vi "FPGA.vi"() -> ()   [LabVIEW 2015]
uses:
  <vilib>/Platform/TimedLoop/XDataNode/timing_clust.ctl
  <vilib>/Platform/TimedLoop/XDataNode/nitl_modes.ctl
  <vilib>/Platform/TimedLoop/XDataNode/wakeup.ctl
  <vilib>/rvi/Emulation/niFpgaGetClockAttributes.vi
  <vilib>/rvi/Emulation/niFpgaSctlEmulationGetInTimedLoop.vi
  <vilib>/rvi/Emulation/niFpgaEmulationReportErrorSimple.vi
  <vilib>/rvi/eio/common/nirviEmuTemplateMethod_errors.vi
  <vilib>/rvi/Emulation/niFpgaCriticalErrorInLSC.vi
  <vilib>/rvi/Emulation/niFpgaEmulationIsFPGAContextNoSignature.vi
  <vilib>/rvi/DataTransferAndStorage/Container/Common/niFpgaContainerGetUniqueNameForEmu.vi
  <vilib>/rvi/Memory/Memory_Emulation/niFpgaMemoryEmulationCacheClearOnFirstRun.vi
  <vilib>/rvi/Memory/Memory_Emulation/nirvimemoryEmulationManagerCache_MakeExclusive.vi
  <vilib>/rvi/Memory/Memory_Emulation/niFpgaMemoryEmulationValidateCache.vi
  <vilib>/rvi/Memory/Memory_Emulation/nirvimemoryEmulationManagerCache_InsertValue.vi
  <vilib>/Utility/error.llb/Clear Errors.vi
  <vilib>/rvi/Memory/Memory_Emulation/nirvimemoryEmulationManagerCache_ReleaseExclusive.vi
  <vilib>/rvi/Memory/Memory_Emulation/nirvimemoryEmulationManagerCache_GetValue.vi
  <vilib>/rvi/Memory/Memory_Emulation/nirvimemoryEmulationManagerCache_SetValue.vi
  <vilib>/rvi/Emulation/niFpgaProcessEmulError.vi
  <vilib>/rvi/Memory/Memory_Emulation/nirvimemoryFastEmulation.vi
  <vilib>/rvi/Memory/Memory_Emulation/nirvimemoryEmulation.vi
  <vilib>/rvi/errors/nirviReportUnexpectedCaseInternalError (U32).vi
  <vilib>/eio/EIONode/EIONode.xnode
  <vilib>/Platform/TimedLoop/XDataNode/XDataNode.xnode
  <vilib>/rvi/DataTransferAndStorage/Container/XNode/niFpgaContainer.xnode
  <vilib>/rvi/DataTransferAndStorage/Register/Emulation/niFpgaRegisterEmulation.vi
  <vilib>/Platform/TimedLoop/XDataNode/XDNodeRunTimeDep.lvlib
panel:
  in  "Амплитуда (0-4096)":u16=4096
  out "Принимаемые\nданные":u16[](array[numeric]) format="%04x"
  out "Ошибка \nпередачи на ОУ":bool
  out "Ошибка \nчтения из ОУ":bool
  in  "RX":bool
  out "TX":bool
  in  "Передаваемые данные":u16[](array[numeric])=[4, 821, 65535, 13380, 0, 0, 0, 0, 0, 0, 0, 0, 0, 0, 0, 0, 0, 0, 0, 0, 0, 0, 0, 0, 0, 0, 0, 0, 0, 0, 0, 0, 0, 0] format="%04x"
  in  "Кол-во слов \nдля приема":u8=4
  in  "Кол-во слов \nдля передачи":u8=1
  in  "адрес ОУ (0-30)":u8=8
  in  "Подадрес (1-30)":u8=4
  in  "Команда управления":T1(ring)=enum."Блокировать передатчик"
  in  "Отправить\nRx CMD":bool
  in  "Отправить\nTx CMD":bool
  in  "Отправить команду ОУ":bool
  out "Машина состояний КШ":T2
  # "Тестовая панель контроллера шины  MIL STD 1553"
  # "Настройки"
  # "Команда передачи:"
  # "Управление ОУ:"
  # "Команда чтения:"
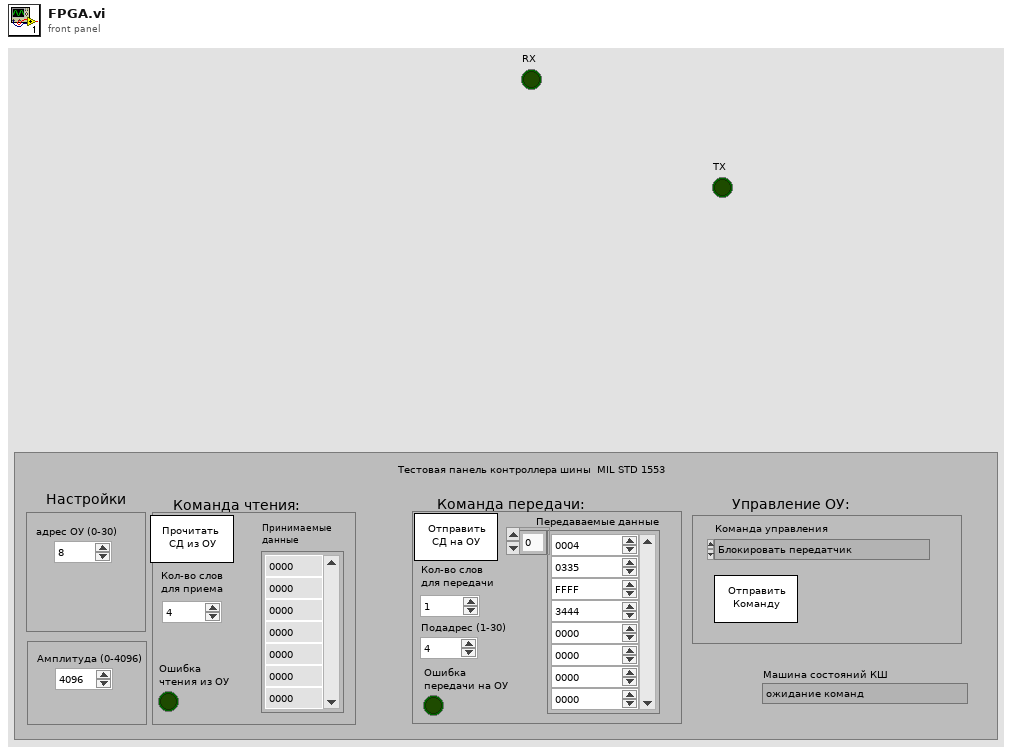
[diagram p1: front panel]
types:
  T1 = enum16{"Принять управление интерфейсом", "Синхронизация", "Передать ОС", "Начать самоконтроль ОУ", "Блокировать передатчик", "Разблокировать передатчик", "Блокировать признак неисправности ОУ", "Разблокировать признак неисправнотси ОУ", "Установить ОУ в исходное состояние", "Резерв", "Передать векорное слово", "Синхронизвция с СД", "Передать последнюю команду", "Передать слово ВСК ОУ", "Блокировать i-й передатчик", "Разблокировать i-й передатчик", "Резерв 2"}
  T2 = typedef "машина состояний КШ.ctl" = enum16{"ожидание команд", "Подготовка команды RX", "Подготовка команды TX", "кодер манчестер КС", "таймаут t2 между словами", "Передача", "ожидание rising СД", "замер длительности true СД", "чтение бит СД", "манчестер декодер СД", "чтение СД", "ожидание rising ОС", "замер длительности false ОС", "замер длительности true OC", "чтение бит ОС", "манчестер декодер ОС", "чтение ОС", "подготовка СД", "кодирование СД", "отправка СД"}
  T3 = typedef "XDNodeRunTimeDep.lvlib/timing_clust.ctl" = cluster{"Expected End [f-1]":u64, "Actual End [f-1]":u64, "Finished Late? [f-1]":bool, "Expected End [i-1]":u64, "Actual End [i-1]":u64, "Finished Late? [i-1]":bool, "Expected Start [i]":u64, "Actual Start [i]":u64, "Expected Start [f]":u64, "Actual Start [f]":u64, "Source Name":string, "Structure Name":string, "Period":i64, "Deadline":i64, "Offset":i64, "Start":i64, "Priority":i32, "Timeout":i32, "Mode":T4, "Wakeup Reason":T5, "Error":errorcluster, "Source Type":string, "Secondary Source Type":string, "Global End Time":u64, "Global Start Time":u64, "Frame Duration":u64, "Iteration Duration":u64, "Assigned CPU":i32, "I/O Scan Engine Mode":u32}
  T4 = typedef "XDNodeRunTimeDep.lvlib/nitl_modes.ctl" = enum32{"No Change", "Process missed periods, maintain original phase", "Discard missed periods, maintain original phase", "Process missed periods, ignore original phase", "Discard missed periods, ignore original phase"}
  T5 = typedef "XDNodeRunTimeDep.lvlib/wakeup.ctl" = enum32{"Normal", "Aborted", "Asynchronous wakeup", "Timing source error", "Timed loop error", "Timeout"}
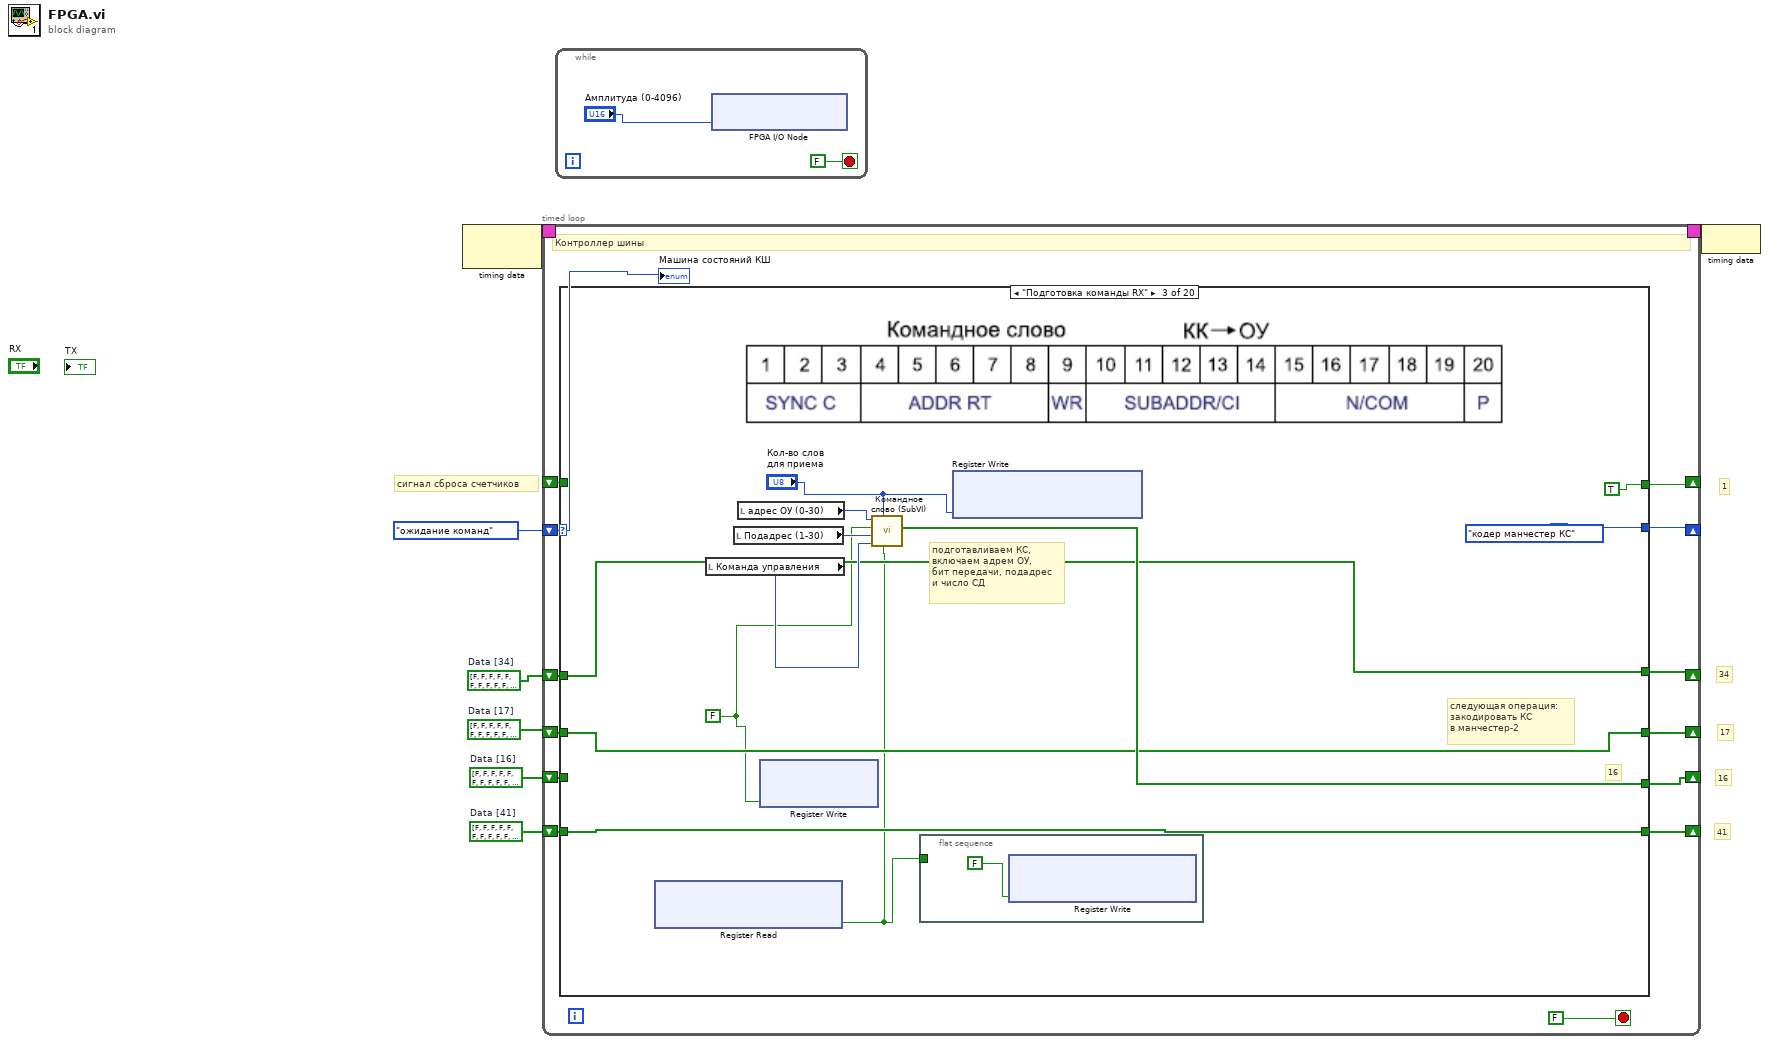
[diagram p0: block diagram]
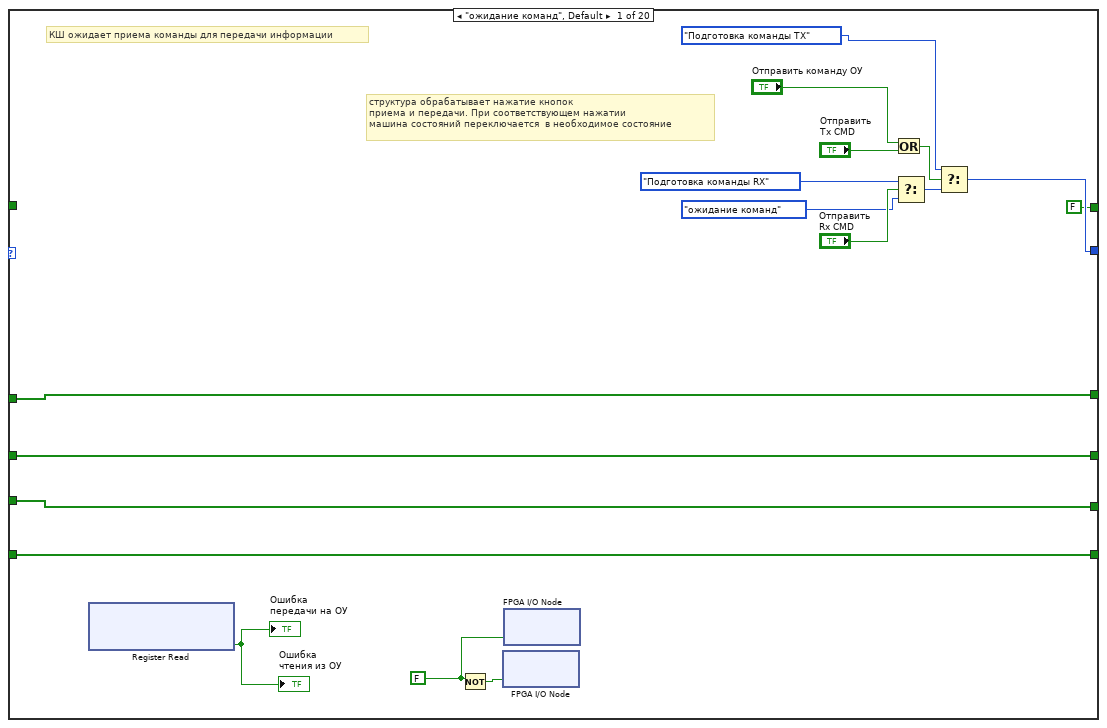
[diagram p2: hidden frame]
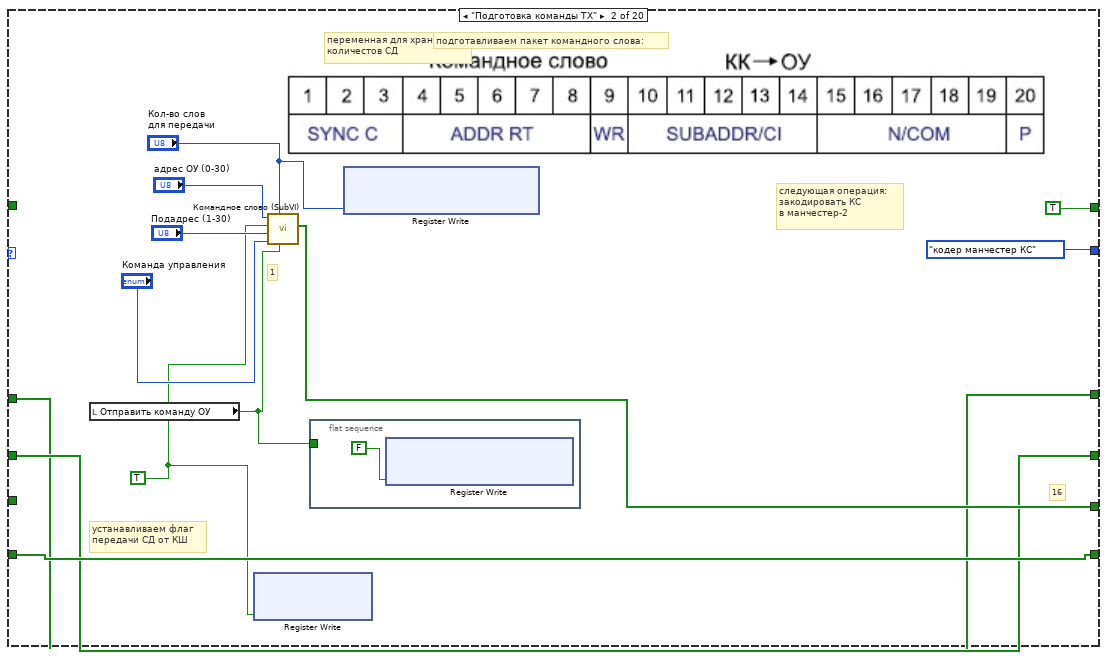
[diagram p3: hidden frame]
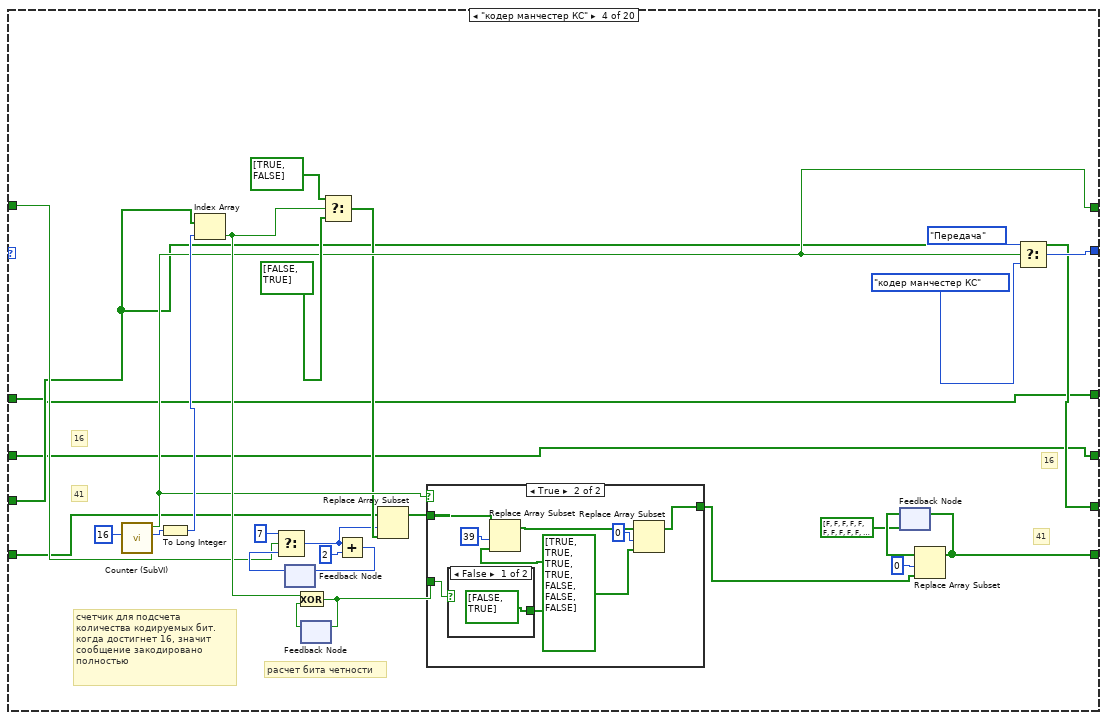
[diagram p4: hidden frame]
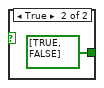
[diagram p6: hidden frame]
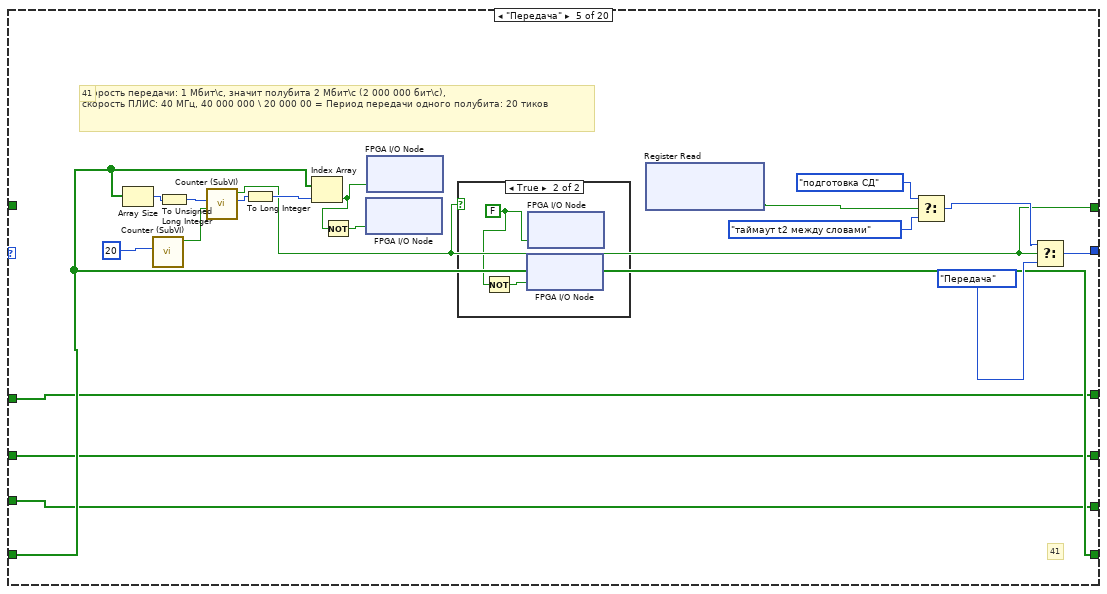
[diagram p7: hidden frame]
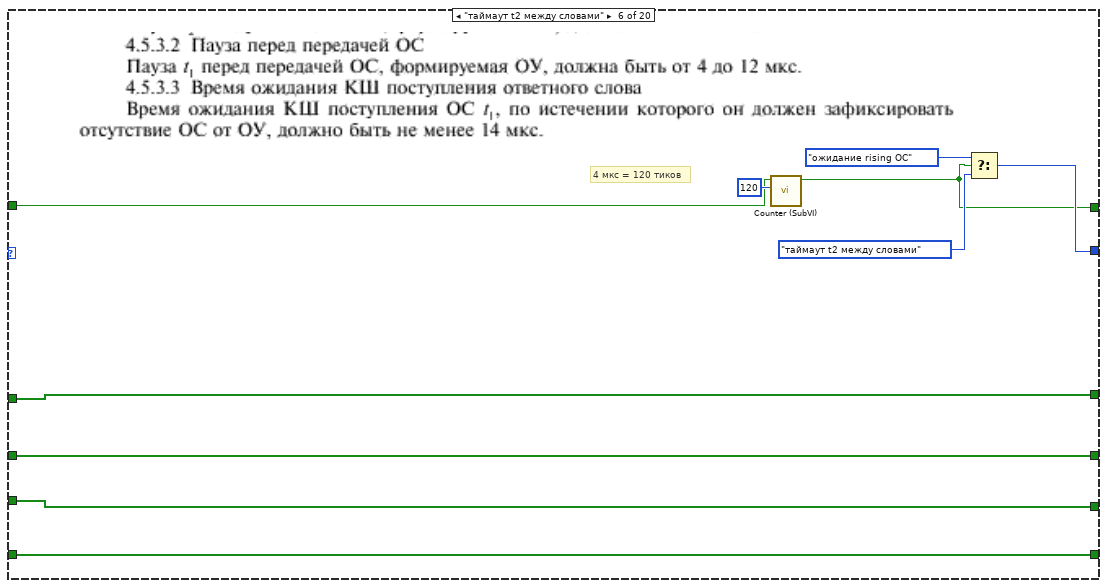
[diagram p9: hidden frame]
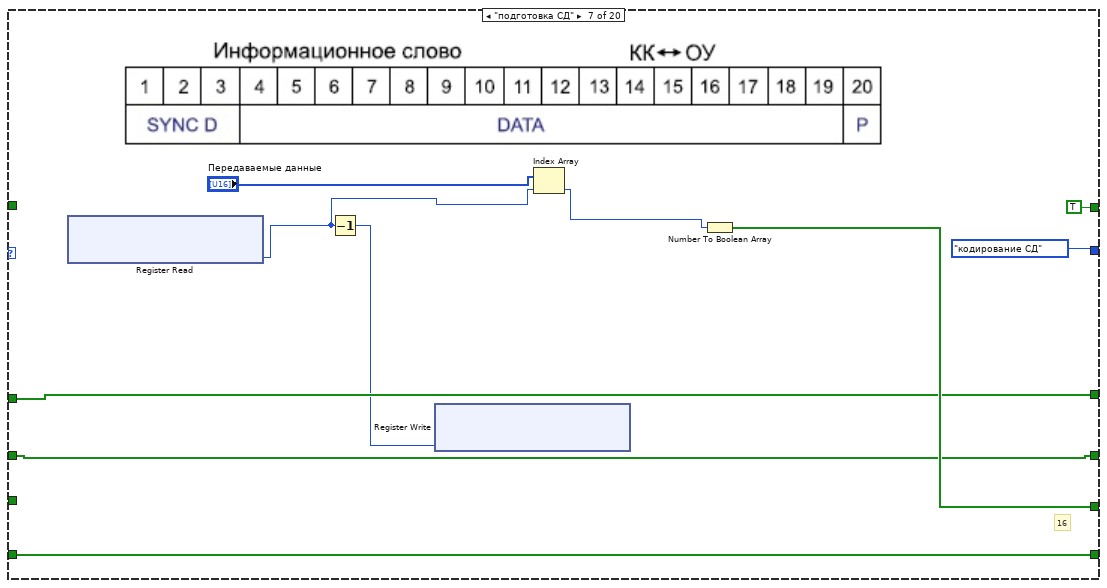
[diagram p10: hidden frame]
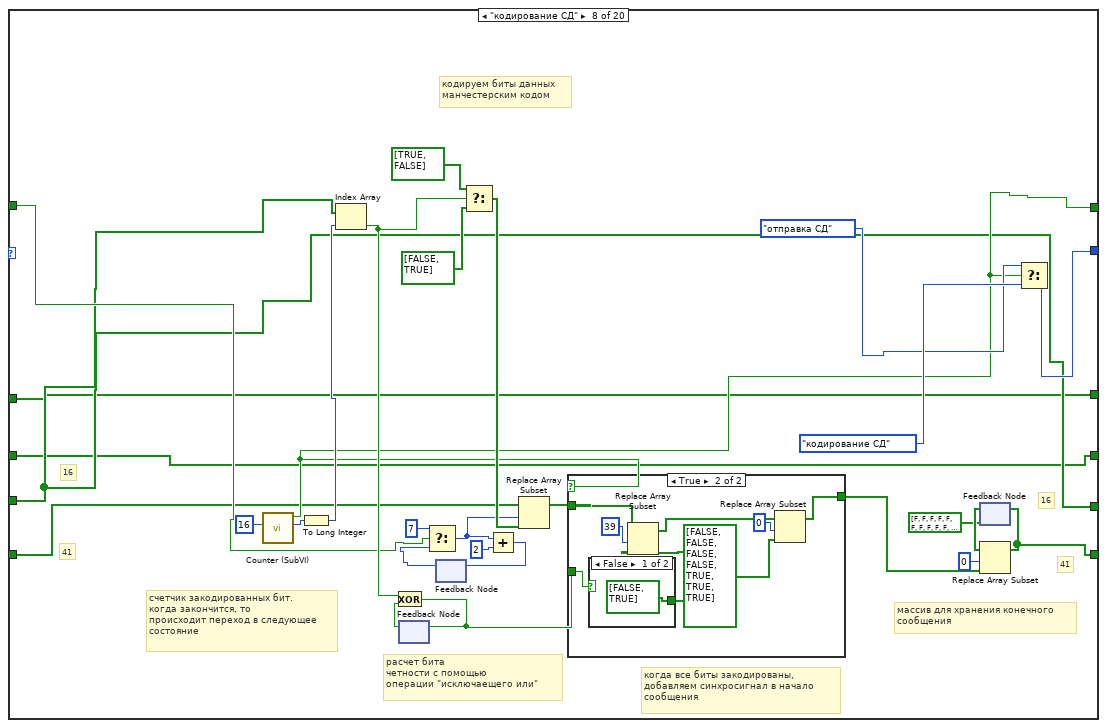
[diagram p11: hidden frame]
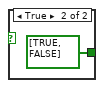
[diagram p13: hidden frame]
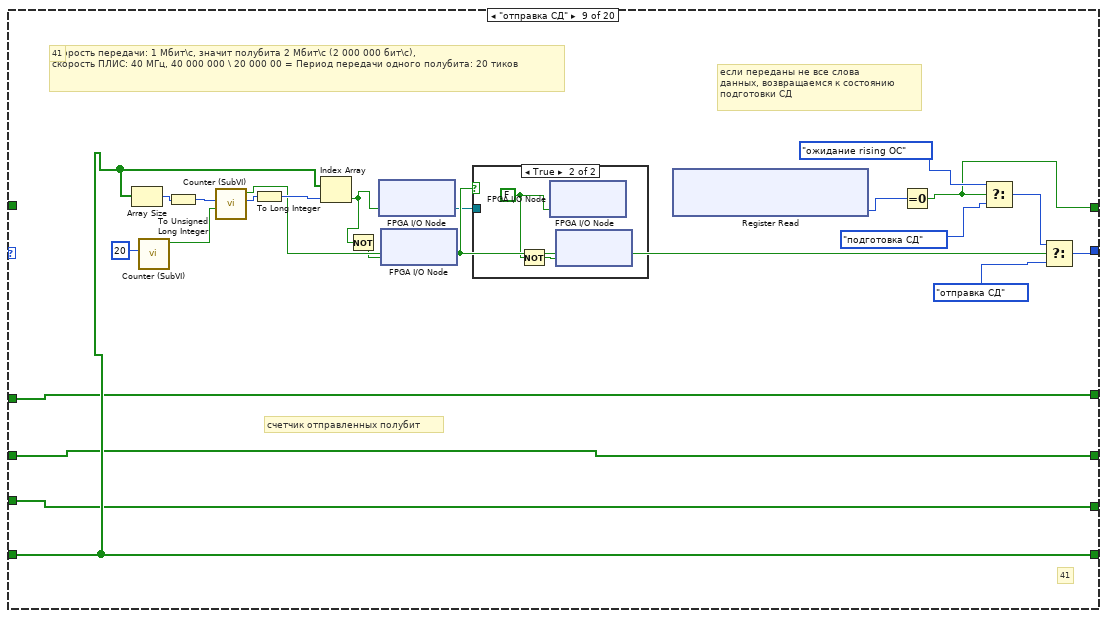
[diagram p14: hidden frame]
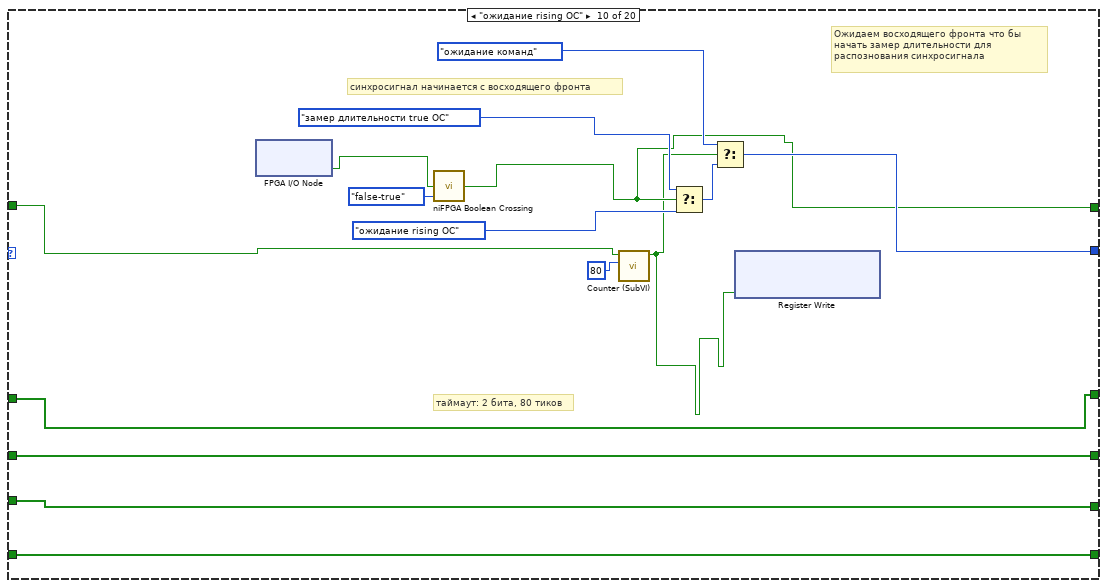
[diagram p16: hidden frame]
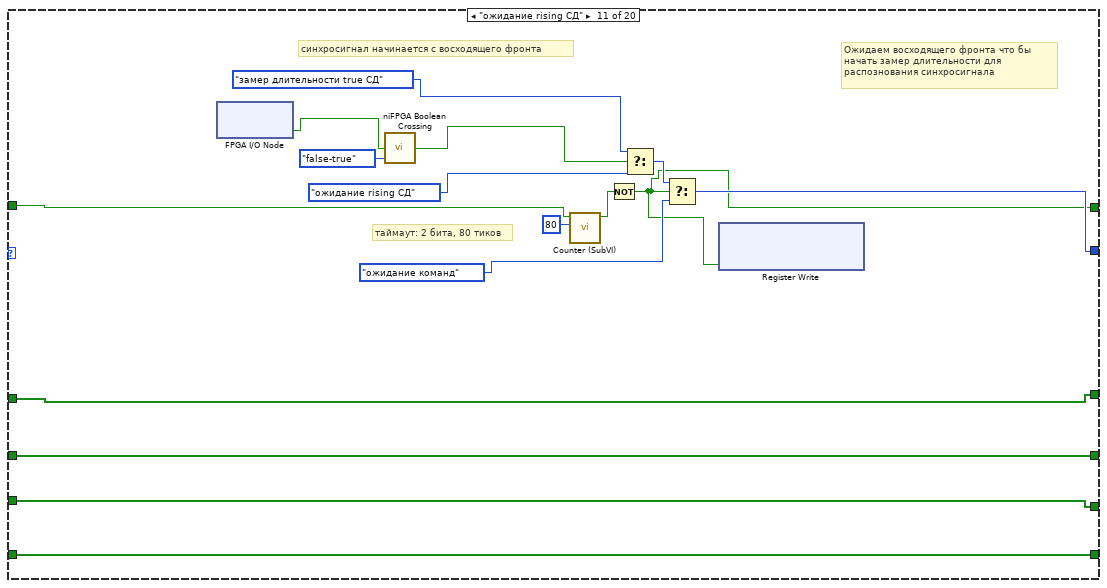
[diagram p17: hidden frame]
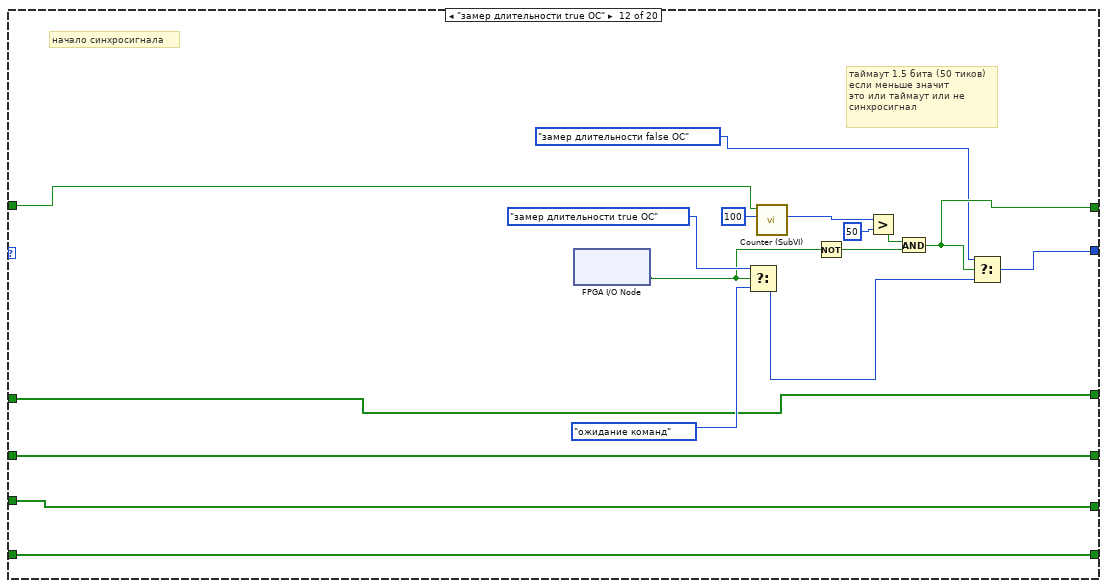
[diagram p18: hidden frame]
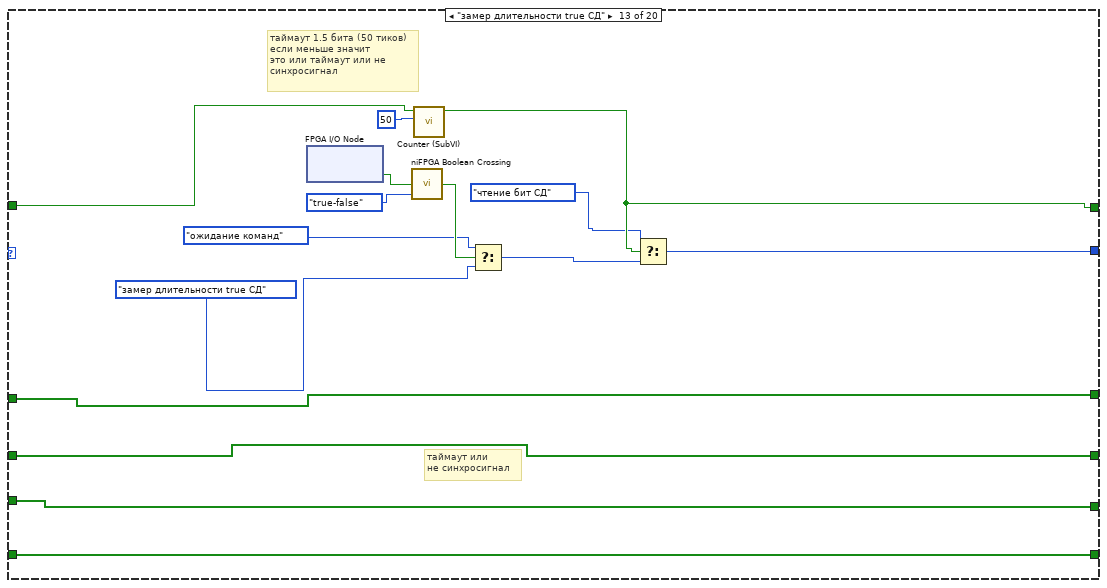
[diagram p19: hidden frame]
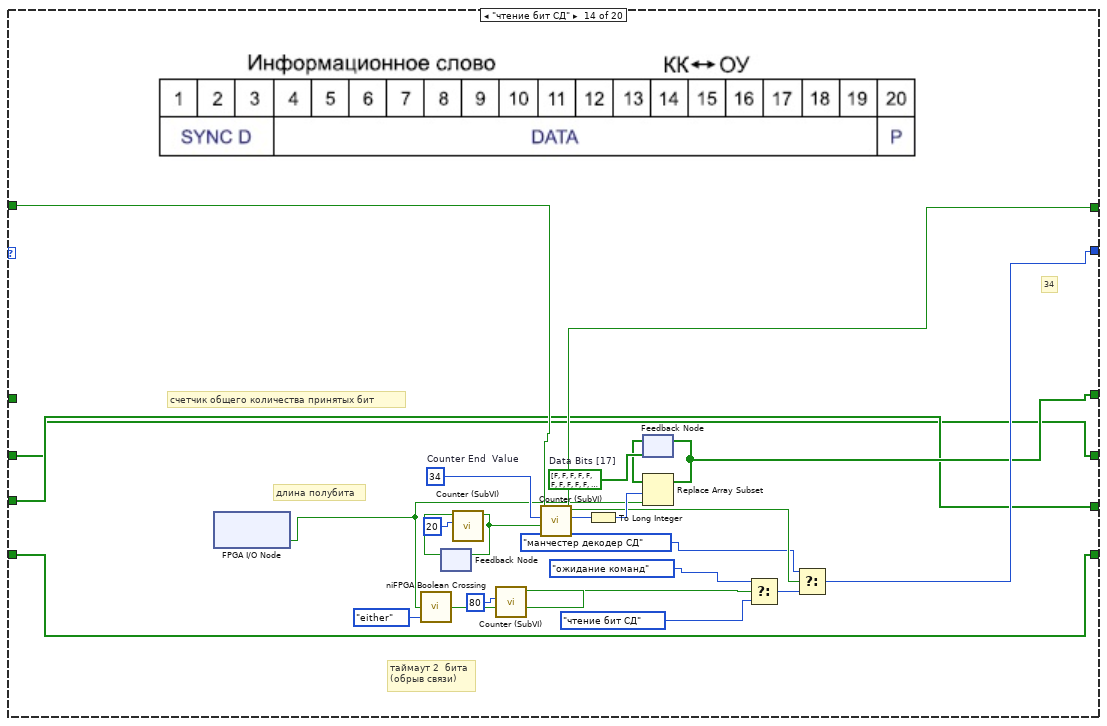
[diagram p20: hidden frame]
diagram:
  w3 = bool[] [FALSE, FALSE, FALSE, FALSE, FALSE, FALSE, FALSE, FALSE, FALSE, FALSE, FALSE, FALSE, FALSE, FALSE, FALSE, FALSE, FALSE, FALSE, FALSE, FALSE, FALSE, FALSE, FALSE, FALSE, FALSE, FALSE, FALSE, FALSE, FALSE, FALSE, FALSE, FALSE, FALSE, FALSE, FALSE, FALSE, FALSE, FALSE, FALSE, FALSE, FALSE]  # Data [41]
  w4 = bool[] [FALSE, FALSE, FALSE, FALSE, FALSE, FALSE, FALSE, FALSE, FALSE, FALSE, FALSE, FALSE, FALSE, FALSE, FALSE, FALSE]  # Data [16]
  w5 = bool[] [FALSE, FALSE, FALSE, FALSE, FALSE, FALSE, FALSE, FALSE, FALSE, FALSE, FALSE, FALSE, FALSE, FALSE, FALSE, FALSE, FALSE]  # Data [17]
  w6 = bool[] [FALSE, FALSE, FALSE, FALSE, FALSE, FALSE, FALSE, FALSE, FALSE, FALSE, FALSE, FALSE, FALSE, FALSE, FALSE, FALSE, FALSE, FALSE, FALSE, FALSE, FALSE, FALSE, FALSE, FALSE, FALSE, FALSE, FALSE, FALSE, FALSE, FALSE, FALSE, FALSE, FALSE, FALSE]  # Data [34]
  # "1"
  # "34"
  # "41"
  # "17"
  # "16"
  # "сигнал сброса счетчиков"
  n1 = node-c288() -> (w2:T3)  [unwired: 1 in]
  n2 = timed-loop {
    shift-right: [w19] -> _
    shift-left: машина_состояний_КШ."ожидание команд" ("Машина состояний КШ") -> [w12]
    shift-right: [w18] -> _
    shift-left: _ -> [w17]
    shift-right: [w16] -> _
    shift-left: w6 -> [w15]
    shift-right: [w14] -> _
    shift-left: w5 -> [w13]
    shift-right: [w8] -> _
    shift-left: w4 -> [w10]
    shift-right: [w9] -> _
    shift-left: w3 -> [w11]
    timing: w2 -> [_]
    timing-out: [_] -> w1
    stop <- FALSE stop-if-true
    # "Контроллер шины"
    n3 = case shown="\"Подготовка команды RX\"" w12 {
      tunnel: [w36 машина_состояний_КШ."кодер манчестер КС" ("Машина состояний КШ") машина_состояний_КШ."кодер манчестер КС" ("Машина состояний КШ") w83 w118 w133 машина_состояний_КШ."кодирование СД" ("Машина состояний КШ") w162 w194 w221 w235 w249 w264 w280 w316 w338 w349 w362 w400 w416] -> w19
      tunnel: [FALSE ("End Reached") TRUE ("End Reached") TRUE ("End Reached") w80 w111 w129 TRUE ("End Reached") w150 w193 w215 w223 w248 w265 w281 FALSE ("End Reached") FALSE ("End Reached") w348 w364 FALSE ("End Reached") FALSE ("End Reached")] -> w18
      tunnel: w17 -> [_ _ _ w70 _ w130 _ w152 _ w214 w233 w250 w266 w279 w307 _ w350 w365 w392 _]
      tunnel: [w25 w40 w54 w65 w107 w128 w139 w145 w189 w210 w226 w240 w257 w278 w312 w329 w341 w363 w387 w410] -> w16
      tunnel: w15 -> [w25 w40 w54 w65 w107 w128 w139 w145 w189 w210 w226 w240 w257 _ w312 w329 w341 _ w387 w410]
      tunnel: [w26 w41 w55 w64 w108 w127 w140 w146 w190 w211 w227 w241 w258 w272 w315 w330 w342 w356 w399 w411] -> w14
      tunnel: w13 -> [w26 w41 w55 w64 w108 w127 w140 w146 w190 w211 w227 w241 w258 w272 _ w330 w342 w356 _ w411]
      tunnel: w11 -> [w28 w42 w56 w67 w110 w125 w141 w149 w192 w213 w229 w243 w260 w274 w306 w332 w344 w358 w391 w413]
      tunnel: w10 -> [w27 _ _ w66 w109 w126 _ w147 w191 w212 w228 w242 w259 w273 w305 w331 w343 w357 w390 w412]
      tunnel: [w28 w42 w56 w68 w110 w125 w141 w148 w192 w213 w229 w243 w260 w274 w306 w332 w344 w358 w391 w413] -> w9
      tunnel: [w27 w43 w57 w66 w109 w126 w142 w147 w191 w212 w228 w242 w259 w273 w305 w331 w343 w357 w390 w412] -> w8
      frame "ожидание команд", Default {
        w21 = FALSE ("TX")
        # "структура обрабатывает нажатие кнопок \nприема и передачи. При соответствующем нажатии\nмашина состояний переключается  в необходимое состояние"
        # "КШ ожидает приема команды для передачи информации"
        n4 = xnode ("Register Read")() -> ("Data"=→"Ошибка \nчтения из ОУ" →"Ошибка \nпередачи на ОУ":bool)  [unwired: 1 in, 1 out]
        n5 = Not(x=w21) -> (.not. x?=w22:bool)
        n6 = xnode "FPGA I/O Node"("TXinv"=w22) -> ()  [unwired: 1 in, 1 out]
        n7 = xnode "FPGA I/O Node"("TX"=w21) -> ()  [unwired: 1 in, 1 out]
        n8 = Or(x="Отправить команду ОУ", y="Отправить\nTx CMD") -> (x .or. y?=w32:bool)
        n9 = Select(t=машина_состояний_КШ."Подготовка команды RX" ("Машина состояний КШ"), s="Отправить\nRx CMD", f=машина_состояний_КШ."ожидание команд" ("Машина состояний КШ")) -> (s? t:f=w35:T2)
        n10 = Select(t=машина_состояний_КШ."Подготовка команды TX" ("Машина состояний КШ"), s=w32, f=w35) -> (s? t:f=w36:T2)
      }
      frame "Подготовка команды TX" {
        w39 = TRUE ("Разряд прием\\передача")
        # "16"
        # "устанавливаем флаг\nпередачи СД от КШ"
        # "следующая операция:\nзакодировать КС\nв манчестер-2"
        # "переменная для хранения\nколичестов СД"
        # "1"
        # "подготавливаем пакет командного слова:"
        n11 = local read "Отправить команду ОУ"() -> (w46:bool)
        n12 = xnode ("Register Write")("Data"=w39) -> ()  [unwired: 1 in, 1 out]
        n13 = call "Командное слово (SubVI).vi"("Признак команды"=w46, "Кол-во слов (1-32)"="Кол-во слов \nдля передачи", "Команда управления"="Команда управления", "Подадрес (1-30)"="Подадрес (1-30)", "Разряд прием\\передача"=w39, "адрес ОУ (0-30)"="адрес ОУ (0-30)") -> ("КС"=w43:bool[])  [unwired: 5 in]
        n14 = flat-sequence {
          tunnel: w46 -> [_]
          frame #0 {
            n15 = xnode ("Register Write")("Data"=FALSE ("Отправить команду ОУ")) -> ()  [unwired: 1 in, 1 out]
          }
        }
        n16 = xnode ("Register Write")("Data"="Кол-во слов \nдля передачи") -> ()  [unwired: 1 in, 1 out]
      }
      frame "Подготовка команды RX" {
        w53 = FALSE ("Разряд прием\\передача 2")
        # "16"
        # "следующая операция:\nзакодировать КС\nв манчестер-2"
        # "подготавливаем КС,\nвключаем адрем ОУ,\nбит передачи, подадрес\nи число СД"
        n17 = xnode ("Register Read")() -> ("Data"=w52:bool)  [unwired: 1 in, 1 out]
        n18 = local read "Команда управления"() -> (w60:T1)
        n19 = local read "Подадрес (1-30)"() -> (w61:u8)
        n20 = local read "адрес ОУ (0-30)"() -> (w62:u8)
        n21 = xnode ("Register Write")("Data"=w53) -> ()  [unwired: 1 in, 1 out]
        n22 = call "Командное слово (SubVI).vi"("Признак команды"=w52, "Кол-во слов (1-32)"="Кол-во слов \nдля приема", "Команда управления"=w60, "Подадрес (1-30)"=w61, "Разряд прием\\передача"=w53, "адрес ОУ (0-30)"=w62) -> ("КС"=w57:bool[])  [unwired: 5 in]
        n23 = flat-sequence {
          tunnel: w52 -> [_]
          frame #0 {
            n24 = xnode ("Register Write")("Data"=FALSE ("Отправить команду ОУ")) -> ()  [unwired: 1 in, 1 out]
          }
        }
        n25 = xnode ("Register Write")("Data"="Кол-во слов \nдля приема") -> ()  [unwired: 1 in, 1 out]
      }
      frame "кодер манчестер КС" {
        # "16"
        # "41"
        # "41"
        # "16"
        # "расчет бита четности"
        # "счетчик для подсчета\nколичества кодируемых бит.\nкогда достигнет 16, значит\nсообщение закодировано \nполностью"
        n26 = call "Counter (SubVI).vi"("Counter End  Value"=u32 16) -> ("Counter Value"=w86:u32, "End Reached"=w80:bool)  [unwired: 9 in]
        n27 = To Long Integer(number=w86) -> (32bit integer=w89:i32)
        n28 = Index Array(array=w66, index=w89) -> (element=w91:bool)
        n29 = feedback #1() -> (w72:i32)  [unwired: 1 in]
        n30 = Select(t=7 ("length"), s=w70, f=w72) -> (s? t:f=w69:i32)
        n31 = feedback #2() -> (w90:bool)  [unwired: 1 in]
        n32 = Exclusive Or(1:w90, 2:w91) -> (0:w92:bool)
        n33 = feedback-in #2(w92) -> ()
        n34 = Select(t=bool[] [TRUE, FALSE], s=w91, f=bool[] [FALSE, TRUE]) -> (s? t:f=w75:bool[])
        n35 = Add(x=w69, y=2 ("length")) -> (x+y=w73:i32)
        n36 = feedback-in #1(w73) -> ()
        n37 = Replace Array Subset(array=w67, new element=w75, index=w69) -> (w88:bool[])
        n38 = case shown="True" w80 {
          tunnel: w88 -> [w93 w99]
          tunnel: [w93 w100] -> w77
          tunnel: w92 -> [_ w96]
          frame False {
          }
          frame True {
            n39 = case shown="False" w96 {
              tunnel: [bool[] [FALSE, TRUE] bool[] [TRUE, FALSE]] -> w95
              frame False {
              }
              frame True {
              }
            }
            n40 = Replace Array Subset(array=w99, new element=w95, index=39) -> (w98:bool[])
            n41 = Replace Array Subset(array=w98, new element=bool[] [TRUE, TRUE, TRUE, TRUE, FALSE, FALSE, FALSE], index=0) -> (w100:bool[])
          }
        }
        n42 = feedback #3(bool[] [FALSE, FALSE, FALSE, FALSE, FALSE, FALSE, FALSE, FALSE, FALSE, FALSE, FALSE, FALSE, FALSE, FALSE, FALSE, FALSE, FALSE, FALSE, FALSE, FALSE, FALSE, FALSE, FALSE, FALSE, FALSE, FALSE, FALSE, FALSE, FALSE, FALSE, FALSE, FALSE, FALSE, FALSE, FALSE, FALSE, FALSE, FALSE, FALSE, FALSE, FALSE]) -> (w79:bool[])
        n43 = Replace Array Subset(array=w79, new element=w77, index=0) -> (w68:bool[])
        n44 = feedback-in #3(w68) -> ()
        n45 = Select(t=машина_состояний_КШ."Передача" ("Машина состояний КШ"), s=w80, f=машина_состояний_КШ."кодер манчестер КС" ("Машина состояний КШ")) -> (s? t:f=w83:T2)
      }
      frame "Передача" {
        # "скорость передачи: 1 Мбит\\с, значит полубита 2 Мбит\\с (2 000 000 бит\\с),\nскорость ПЛИС: 40 МГц, 40 000 000 \\ 20 000 00 = Период передачи одного полубита: 20 тиков"
        # "41"
        # "41"
        n46 = Array Size(array=w110) -> (size(s)=w116:i32)
        n47 = call "Counter (SubVI).vi"("Counter End  Value"=u32 20) -> ("End Reached"=w119:bool)  [unwired: 9 in, 1 out]
        n48 = To Unsigned Long Integer(number=w116) -> (unsigned 32bit integer=w115:u32)
        n49 = call "Counter (SubVI).vi"("Input Valid"=w119, "Counter End  Value"=w115) -> ("Counter Value"=w122:u32, "End Reached"=w111:bool)  [unwired: 8 in]
        n50 = To Long Integer(number=w122) -> (32bit integer=w121:i32)
        n51 = Index Array(array=w110, index=w121) -> (element=w104:bool)
        n52 = Not(x=w104) -> (.not. x?=w105:bool)
        n53 = xnode "FPGA I/O Node"("TXinv"=w105) -> ()  [unwired: 1 in, 1 out]
        n54 = xnode "FPGA I/O Node"("TX"=w104) -> ()  [unwired: 1 in, 1 out]
        n55 = case shown="True" w111 {
          frame False {
          }
          frame True {
            w123 = FALSE ("TX")
            n56 = Not(x=w123) -> (.not. x?=w124:bool)
            n57 = xnode "FPGA I/O Node"("TXinv"=w124) -> ()  [unwired: 1 in, 1 out]
            n58 = xnode "FPGA I/O Node"("TX"=w123) -> ()  [unwired: 1 in, 1 out]
          }
        }
        n59 = xnode ("Register Read")() -> ("Data"=w106:bool)  [unwired: 1 in, 1 out]
        n60 = Select(t=машина_состояний_КШ."подготовка СД" ("Машина состояний КШ"), s=w106, f=машина_состояний_КШ."таймаут t2 между словами" ("Машина состояний КШ")) -> (s? t:f=w113:T2)
        n61 = Select(t=w113, s=w111, f=машина_состояний_КШ."Передача" ("Машина состояний КШ")) -> (s? t:f=w118:T2)
      }
      frame "таймаут t2 между словами" {
        # "4 мкс = 120 тиков"
        n62 = call "Counter (SubVI).vi"("Counter End  Value"=u32 120, "Reset"=w130) -> ("End Reached"=w129:bool)  [unwired: 8 in, 1 out]
        n63 = Select(t=машина_состояний_КШ."ожидание rising ОС" ("Машина состояний КШ"), s=w129, f=машина_состояний_КШ."таймаут t2 между словами" ("Машина состояний КШ")) -> (s? t:f=w133:T2)
      }
      frame "подготовка СД" {
        # "16"
        n64 = xnode ("Register Read")() -> ("Data"=w136:u8)  [unwired: 1 in, 1 out]
        n65 = Decrement(x=w136) -> (x-1=w138:u8)
        n66 = xnode ("Register Write")("Data"=w138) -> ()  [unwired: 1 in, 1 out]
        n67 = Index Array(array="Передаваемые данные", index=w136) -> (element=w135:u16)
        n68 = Number To Boolean Array(number=w135) -> (Boolean array=w142:bool[])
      }
      frame "кодирование СД" {
        # "массив для хранения конечного\nсообщения"
        # "кодируем биты данных\nманчестерским кодом"
        # "когда все биты закодированы,\nдобавляем синхросигнал в начало \nсообщения"
        # "расчет бита\nчетности с помощью\nоперации \"исключаещего или\""
        # "счетчик закодированных бит.\nкогда закончится, то \nпроисходит переход в следующее\nсостояние"
        # "16"
        # "41"
        # "41"
        # "16"
        n69 = call "Counter (SubVI).vi"("Counter End  Value"=u32 16) -> ("Counter Value"=w167:u32, "End Reached"=w150:bool)  [unwired: 9 in]
        n70 = To Long Integer(number=w167) -> (32bit integer=w170:i32)
        n71 = Index Array(array=w147, index=w170) -> (element=w172:bool)
        n72 = feedback #4() -> (w171:bool)  [unwired: 1 in]
        n73 = Exclusive Or(1:w171, 2:w172) -> (0:w173:bool)
        n74 = feedback-in #4(w173) -> ()
        n75 = feedback #5() -> (w156:i32)  [unwired: 1 in]
        n76 = Select(t=7 ("length"), s=w152, f=w156) -> (s? t:f=w151:i32)
        n77 = Select(t=bool[] [TRUE, FALSE], s=w172, f=bool[] [FALSE, TRUE]) -> (s? t:f=w157:bool[])
        n78 = Add(x=w151, y=2 ("length")) -> (x+y=w154:i32)
        n79 = feedback-in #5(w154) -> ()
        n80 = Replace Array Subset(array=w149, new element=w157, index=w151) -> (w169:bool[])
        n81 = case shown="True" w150 {
          tunnel: w169 -> [w174 w180]
          tunnel: [w174 w181] -> w158
          tunnel: w173 -> [_ w177]
          frame False {
          }
          frame True {
            n82 = case shown="False" w177 {
              tunnel: [bool[] [FALSE, TRUE] bool[] [TRUE, FALSE]] -> w176
              frame False {
              }
              frame True {
              }
            }
            n83 = Replace Array Subset(array=w180, new element=w176, index=39) -> (w179:bool[])
            n84 = Replace Array Subset(array=w179, new element=bool[] [FALSE, FALSE, FALSE, FALSE, TRUE, TRUE, TRUE], index=0) -> (w181:bool[])
          }
        }
        n85 = feedback #6(bool[] [FALSE, FALSE, FALSE, FALSE, FALSE, FALSE, FALSE, FALSE, FALSE, FALSE, FALSE, FALSE, FALSE, FALSE, FALSE, FALSE, FALSE, FALSE, FALSE, FALSE, FALSE, FALSE, FALSE, FALSE, FALSE, FALSE, FALSE, FALSE, FALSE, FALSE, FALSE, FALSE, FALSE, FALSE, FALSE, FALSE, FALSE, FALSE, FALSE, FALSE, FALSE]) -> (w161:bool[])
        n86 = Replace Array Subset(array=w161, new element=w158, index=0) -> (w148:bool[])
        n87 = feedback-in #6(w148) -> ()
        n88 = Select(t=машина_состояний_КШ."отправка СД" ("Машина состояний КШ"), s=w150, f=машина_состояний_КШ."кодирование СД" ("Машина состояний КШ")) -> (s? t:f=w162:T2)
      }
      frame "отправка СД" {
        # "если переданы не все слова\nданных, возвращаемся к состоянию\nподготовки СД"
        # "счетчик отправленных полубит"
        # "скорость передачи: 1 Мбит\\с, значит полубита 2 Мбит\\с (2 000 000 бит\\с),\nскорость ПЛИС: 40 МГц, 40 000 000 \\ 20 000 00 = Период передачи одного полубита: 20 тиков"
        # "41"
        # "41"
        n89 = Array Size(array=w192) -> (size(s)=w198:i32)
        n90 = call "Counter (SubVI).vi"("Counter End  Value"=u32 20) -> ("End Reached"=w200:bool)  [unwired: 9 in, 1 out]
        n91 = To Unsigned Long Integer(number=w198) -> (unsigned 32bit integer=w197:u32)
        n92 = call "Counter (SubVI).vi"("Input Valid"=w200, "Counter End  Value"=w197) -> ("Counter Value"=w203:u32, "End Reached"=w196:bool)  [unwired: 8 in]
        n93 = To Long Integer(number=w203) -> (32bit integer=w202:i32)
        n94 = Index Array(array=w192, index=w202) -> (element=w185:bool)
        n95 = Not(x=w185) -> (.not. x?=w186:bool)
        n96 = xnode "FPGA I/O Node"("TX"=w185) -> ("FPGA I/O Out"=w187:refnum<k21>)  [unwired: 1 in]
        n97 = xnode "FPGA I/O Node"("TXinv"=w186) -> ()  [unwired: 1 in, 1 out]
        n98 = case shown="True" w196 {
          tunnel: w187 -> [_ _]
          frame False {
          }
          frame True {
            w206 = FALSE ("TX")
            n99 = Not(x=w206) -> (.not. x?=w207:bool)
            n100 = xnode "FPGA I/O Node"("TX"=w206) -> ()  [unwired: 1 in, 1 out]
            n101 = xnode "FPGA I/O Node"("TXinv"=w207) -> ()  [unwired: 1 in, 1 out]
          }
        }
        n102 = xnode ("Register Read")() -> ("Data"=w188:u8)  [unwired: 1 in, 1 out]
        n103 = Equal To 0?(x=w188) -> (x = 0?=w193:bool)
        n104 = Select(t=машина_состояний_КШ."ожидание rising ОС" ("Машина состояний КШ"), s=w193, f=машина_состояний_КШ."подготовка СД" ("Машина состояний КШ")) -> (s? t:f=w195:T2)
        n105 = Select(t=w195, s=w196, f=машина_состояний_КШ."отправка СД" ("Машина состояний КШ")) -> (s? t:f=w194:T2)
      }
      frame "ожидание rising ОС" {
        # "Ожидаем восходящего фронта что бы\nначать замер длительности для \nраспознования синхросигнала"
        # "таймаут: 2 бита, 80 тиков"
        # "синхросигнал начинается с восходящего фронта"
        n106 = xnode "FPGA I/O Node"() -> ("RX"=w209:bool)  [unwired: 1 in, 1 out]
        n107 = call "niFPGA Boolean Crossing.vi"("input"=w209, "direction"=enum8{"either", "false-true", "true-false"}."false-true") -> ("crossing"=w215:bool)  [unwired: 7 in]
        n108 = call "Counter (SubVI).vi"("Counter End  Value"=u32 80, "Reset"=w214) -> ("End Reached"=w208:bool)  [unwired: 8 in, 1 out]
        n109 = Select(t=машина_состояний_КШ."замер длительности true OC" ("Машина состояний КШ"), s=w215, f=машина_состояний_КШ."ожидание rising ОС" ("Машина состояний КШ")) -> (s? t:f=w219:T2)
        n110 = Select(t=машина_состояний_КШ."ожидание команд" ("Машина состояний КШ"), s=w208, f=w219) -> (s? t:f=w221:T2)
        n111 = xnode ("Register Write")("Data"=w208) -> ()  [unwired: 1 in, 1 out]
      }
      frame "ожидание rising СД" {
        # "Ожидаем восходящего фронта что бы\nначать замер длительности для \nраспознования синхросигнала"
        # "таймаут: 2 бита, 80 тиков"
        # "синхросигнал начинается с восходящего фронта"
        n112 = xnode "FPGA I/O Node"() -> ("RX"=w225:bool)  [unwired: 1 in, 1 out]
        n113 = call "niFPGA Boolean Crossing.vi"("input"=w225, "direction"=enum8{"either", "false-true", "true-false"}."false-true") -> ("crossing"=w238:bool)  [unwired: 7 in]
        n114 = call "Counter (SubVI).vi"("Counter End  Value"=u32 80, "Reset"=w233) -> ("End Reached"=w224:bool)  [unwired: 8 in, 1 out]
        n115 = Not(x=w224) -> (.not. x?=w223:bool)
        n116 = Select(t=машина_состояний_КШ."замер длительности true СД" ("Машина состояний КШ"), s=w238, f=машина_состояний_КШ."ожидание rising СД" ("Машина состояний КШ")) -> (s? t:f=w236:T2)
        n117 = Select(t=w236, s=w223, f=машина_состояний_КШ."ожидание команд" ("Машина состояний КШ")) -> (s? t:f=w235:T2)
        n118 = xnode ("Register Write")("Data"=w223) -> ()  [unwired: 1 in, 1 out]
      }
      frame "замер длительности true OC" {
        # "начало синхросигнала"
        # "таймаут 1.5 бита (50 тиков)\nесли меньше значит\nэто или таймаут или не \nсинхросигнал"
        n119 = xnode "FPGA I/O Node"() -> ("RX"=w239:bool)  [unwired: 1 in, 1 out]
        n120 = Select(t=машина_состояний_КШ."замер длительности true OC" ("Машина состояний КШ"), s=w239, f=машина_состояний_КШ."ожидание команд" ("Машина состояний КШ")) -> (s? t:f=w253:T2)
        n121 = call "Counter (SubVI).vi"("Counter End  Value"=u32 100, "Reset"=w250) -> ("Counter Value"=w247:u32)  [unwired: 8 in, 1 out]
        n122 = Not(x=w239) -> (.not. x?=w255:bool)
        n123 = Greater?(x=w247, y=u32 50 ("Counter End  Value")) -> (0:w254:bool)
        n124 = And(x=w254, y=w255) -> (x .and. y?=w248:bool)
        n125 = Select(t=машина_состояний_КШ."замер длительности false ОС" ("Машина состояний КШ"), s=w248, f=w253) -> (s? t:f=w249:T2)
      }
      frame "замер длительности true СД" {
        # "таймаут 1.5 бита (50 тиков)\nесли меньше значит\nэто или таймаут или не \nсинхросигнал"
        # "таймаут или \nне синхросигнал"
        n126 = xnode "FPGA I/O Node"() -> ("RX"=w256:bool)  [unwired: 1 in, 1 out]
        n127 = call "niFPGA Boolean Crossing.vi"("input"=w256, "direction"=enum8{"either", "false-true", "true-false"}."true-false") -> ("crossing"=w270:bool)  [unwired: 7 in]
        n128 = call "Counter (SubVI).vi"("Counter End  Value"=u32 50, "Reset"=w266) -> ("End Reached"=w265:bool)  [unwired: 8 in, 1 out]
        n129 = Select(t=машина_состояний_КШ."ожидание команд" ("Машина состояний КШ"), s=w270, f=машина_состояний_КШ."замер длительности true СД" ("Машина состояний КШ")) -> (s? t:f=w268:T2)
        n130 = Select(t=машина_состояний_КШ."чтение бит СД" ("Машина состояний КШ"), s=w265, f=w268) -> (s? t:f=w264:T2)
      }
      frame "чтение бит СД" {
        w287 = u32 34  # Counter End  Value
        w284 = bool[] [FALSE, FALSE, FALSE, FALSE, FALSE, FALSE, FALSE, FALSE, FALSE, FALSE, FALSE, FALSE, FALSE, FALSE, FALSE, FALSE, FALSE, FALSE, FALSE, FALSE, FALSE, FALSE, FALSE, FALSE, FALSE, FALSE, FALSE, FALSE, FALSE, FALSE, FALSE, FALSE, FALSE, FALSE]  # Data Bits [17]
        # "34"
        # "длина полубита"
        # "счетчик общего количества принятых бит"
        # "таймаут 2  бита\n(обрыв связи)"
        n131 = xnode "FPGA I/O Node"() -> ("RX"=w271:bool)  [unwired: 1 in, 1 out]
        n132 = call "niFPGA Boolean Crossing.vi"("input"=w271, "direction"=enum8{"either", "false-true", "true-false"}."either") -> ("crossing"=w293:bool)  [unwired: 7 in]
        n133 = feedback #7() -> (w290:bool)  [unwired: 1 in]
        n134 = call "Counter (SubVI).vi"("Counter End  Value"=u32 20, "Reset"=w290) -> ("End Reached"=w294:bool)  [unwired: 8 in, 1 out]
        n135 = feedback-in #7(w294) -> ()
        n136 = call "Counter (SubVI).vi"("Counter End  Value"=u32 80, "Reset"=w293) -> ("End Reached"=w292:bool)  [unwired: 8 in, 1 out]
        n137 = call "Counter (SubVI).vi"("Input Valid"=w294, "Counter End  Value"=w287, "Reset"=w279) -> ("Counter Value"=w286:u32, "End Reached"=w281:bool)  [unwired: 7 in]
        n138 = To Long Integer(number=w286) -> (32bit integer=w282:i32)
        n139 = feedback #8(w284) -> (w283:bool[])
        n140 = Replace Array Subset(array=w283, new element=w271, index=w282) -> (w278:bool[])
        n141 = feedback-in #8(w278) -> ()
        n142 = Select(t=машина_состояний_КШ."ожидание команд" ("Машина состояний КШ"), s=w292, f=машина_состояний_КШ."чтение бит СД" ("Машина состояний КШ")) -> (s? t:f=w288:T2)
        n143 = Select(t=машина_состояний_КШ."манчестер декодер СД" ("Машина состояний КШ"), s=w281, f=w288) -> (s? t:f=w280:T2)
      }
      frame "манчестер декодер СД" {
        w319 = bool[] [FALSE, FALSE, FALSE, FALSE, FALSE, FALSE, FALSE, FALSE, FALSE, FALSE, FALSE, FALSE, FALSE, FALSE, FALSE, FALSE, FALSE]  # Data Bits [17]
        # "счетчик раскодированных бит"
        # "Производим сравнение:\nберем два бита по порядку. \nЕсли это истина и ложь, значит \nэто закодирована еденица. \nЗаписываем соответствующее значение\nв масси принимаемых данных"
        # "Эта структура является счетчиком текущего бита."
        # "34"
        # "34"
        # "17"
        n144 = feedback #9() -> (w309:i32)  [unwired: 1 in]
        n145 = Select(t=0 ("length"), s=w307, f=w309) -> (s? t:f=w303:i32)
        n146 = Add(x=w303, y=2 ("length")) -> (x+y=w310:i32)
        n147 = feedback-in #9(w310) -> ()
        n148 = Increment(x=w303) -> (x+1=w302:i32)
        n149 = Index Array(array=w312, index #1=w303, index #2=w302) -> (element #1=w301:bool, element #2=w295:bool)
        n150 = Equal?(x=w301, y=TRUE) -> (x = y?=w298:bool)
        n151 = Equal?(x=w295, y=FALSE) -> (x = y?=w297:bool)
        n152 = And(x=w298, y=w297) -> (x .and. y?=w296:bool)
        n153 = call "Counter (SubVI).vi"("Counter End  Value"=u32 17) -> ("Counter Value"=w320:u32, "End Reached"=w321:bool)  [unwired: 9 in]
        n154 = To Long Integer(number=w320) -> (32bit integer=w317:i32)
        n155 = feedback #10(w319) -> (w318:bool[])
        n156 = Replace Array Subset(array=w318, new element=w296, index=w317) -> (w315:bool[])
        n157 = feedback-in #10(w315) -> ()
        n158 = Select(t=машина_состояний_КШ."чтение СД" ("Машина состояний КШ"), s=w321, f=машина_состояний_КШ."манчестер декодер СД" ("Машина состояний КШ")) -> (s? t:f=w316:T2)
      }
      frame "чтение СД" {
        # "Если счетчик достиг нуля, то транзакция завершена. \nПереходим в ожидания команд. В противном случае \nпереходим в состояние поиска синхросигнала СД."
        # "Уменьшаем счетчик приянытх слов на еденицу"
        # "Преобразуем массив 16 бит в число. \nЗаписываем его в память принимаемых\nданных."
        # "17"
        n159 = xnode ("Register Read")() -> ("Data"=w327:u8)  [unwired: 1 in, 1 out]
        n160 = local read "Принимаемые\nданные"() -> (w326:u16[])
        n161 = Delete From Array(array=w330, length=16, index=0) -> (deleted portion=w333:bool[])  [unwired: 1 out]
        n162 = Boolean Array To Number(Boolean array=w333) -> (number=w323:u32)
        n163 = Decrement(x=w327) -> (x-1=w324:u8)
        n164 = Equal To 0?(x=w324) -> (x = 0?=w339:bool)
        n165 = xnode ("Register Write")("Data"=w324) -> ()  [unwired: 1 in, 1 out]
        n166 = xnode ("Memory Method Node")("Address"=w324, "Data"=w323) -> ()  [unwired: 1 in, 1 out]
        n167 = Replace Array Subset(array=w326, new element=w323, index=w324) -> (→"Принимаемые\nданные":u16[])
        n168 = Select(t=машина_состояний_КШ."ожидание команд" ("Машина состояний КШ"), s=w339, f=машина_состояний_КШ."ожидание rising СД" ("Машина состояний КШ")) -> (s? t:f=w338:T2)
      }
      frame "замер длительности false ОС" {
        # "таймаут 1.5 бита (50 тиков)\nесли меньше значит\nэто или таймаут или не \nсинхросигнал"
        # "таймаут или \nне синхросигнал"
        n169 = xnode "FPGA I/O Node"() -> ("RX"=w340:bool)  [unwired: 1 in, 1 out]
        n170 = call "niFPGA Boolean Crossing.vi"("input"=w340, "direction"=enum8{"either", "false-true", "true-false"}."false-true") -> ("crossing"=w354:bool)  [unwired: 7 in]
        n171 = call "Counter (SubVI).vi"("Counter End  Value"=u32 50, "Reset"=w350) -> ("End Reached"=w348:bool)  [unwired: 8 in, 1 out]
        n172 = Select(t=машина_состояний_КШ."ожидание команд" ("Машина состояний КШ"), s=w354, f=машина_состояний_КШ."замер длительности false ОС" ("Машина состояний КШ")) -> (s? t:f=w352:T2)
        n173 = Select(t=машина_состояний_КШ."чтение бит ОС" ("Машина состояний КШ"), s=w348, f=w352) -> (s? t:f=w349:T2)
      }
      frame "чтение бит ОС" {
        w371 = u32 34  # Counter End  Value
        w368 = bool[] [FALSE, FALSE, FALSE, FALSE, FALSE, FALSE, FALSE, FALSE, FALSE, FALSE, FALSE, FALSE, FALSE, FALSE, FALSE, FALSE, FALSE, FALSE, FALSE, FALSE, FALSE, FALSE, FALSE, FALSE, FALSE, FALSE, FALSE, FALSE, FALSE, FALSE, FALSE, FALSE, FALSE, FALSE]  # Data Bits [17]
        # "34"
        # "длина полубита"
        # "счетчик общего количества принятых бит"
        # "таймаут 2бита\n(обрыв связи)"
        n174 = xnode "FPGA I/O Node"() -> ("RX"=w355:bool)  [unwired: 1 in, 1 out]
        n175 = call "niFPGA Boolean Crossing.vi"("input"=w355, "direction"=enum8{"either", "false-true", "true-false"}."either") -> ("crossing"=w377:bool)  [unwired: 7 in]
        n176 = feedback #11() -> (w374:bool)  [unwired: 1 in]
        n177 = call "Counter (SubVI).vi"("Counter End  Value"=u32 20, "Reset"=w374) -> ("End Reached"=w378:bool)  [unwired: 8 in, 1 out]
        n178 = feedback-in #11(w378) -> ()
        n179 = call "Counter (SubVI).vi"("Counter End  Value"=u32 80, "Reset"=w377) -> ("End Reached"=w376:bool)  [unwired: 8 in, 1 out]
        n180 = call "Counter (SubVI).vi"("Input Valid"=w378, "Counter End  Value"=w371, "Reset"=w365) -> ("Counter Value"=w370:u32, "End Reached"=w364:bool)  [unwired: 7 in]
        n181 = To Long Integer(number=w370) -> (32bit integer=w366:i32)
        n182 = feedback #12(w368) -> (w367:bool[])
        n183 = Replace Array Subset(array=w367, new element=w355, index=w366) -> (w363:bool[])
        n184 = feedback-in #12(w363) -> ()
        n185 = Select(t=машина_состояний_КШ."ожидание команд" ("Машина состояний КШ"), s=w376, f=машина_состояний_КШ."чтение бит ОС" ("Машина состояний КШ")) -> (s? t:f=w372:T2)
        n186 = Select(t=машина_состояний_КШ."манчестер декодер ОС" ("Машина состояний КШ"), s=w364, f=w372) -> (s? t:f=w362:T2)
      }
      frame "манчестер декодер ОС" {
        w403 = bool[] [FALSE, FALSE, FALSE, FALSE, FALSE, FALSE, FALSE, FALSE, FALSE, FALSE, FALSE, FALSE, FALSE, FALSE, FALSE, FALSE, FALSE]  # Data Bits [17]
        # "счетчик раскодированных бит"
        # "Производим сравнение:\nберем два бита по порядку. \nЕсли это истина и ложь, значит \nэто закодирована еденица. \nЗаписываем соответствующее значение\nв масси принимаемых данных"
        # "Эта структура является счетчиком текущего бита."
        # "34"
        # "17"
        # "34"
        n187 = feedback #13() -> (w394:i32)  [unwired: 1 in]
        n188 = Select(t=0 ("length"), s=w392, f=w394) -> (s? t:f=w386:i32)
        n189 = Add(x=w386, y=2 ("length")) -> (x+y=w395:i32)
        n190 = feedback-in #13(w395) -> ()
        n191 = Increment(x=w386) -> (x+1=w388:i32)
        n192 = Index Array(array=w387, index #1=w386, index #2=w388) -> (element #1=w381:bool, element #2=w380:bool)
        n193 = Equal?(x=w381, y=TRUE) -> (x = y?=w383:bool)
        n194 = Equal?(x=w380, y=FALSE) -> (x = y?=w382:bool)
        n195 = call "Counter (SubVI).vi"("Counter End  Value"=u32 17) -> ("Counter Value"=w404:u32, "End Reached"=w405:bool)  [unwired: 9 in]
        n196 = And(x=w383, y=w382) -> (x .and. y?=w379:bool)
        n197 = To Long Integer(number=w404) -> (32bit integer=w401:i32)
        n198 = feedback #14(w403) -> (w402:bool[])
        n199 = Replace Array Subset(array=w402, new element=w379, index=w401) -> (w399:bool[])
        n200 = feedback-in #14(w399) -> ()
        n201 = Select(t=машина_состояний_КШ."чтение ОС" ("Машина состояний КШ"), s=w405, f=машина_состояний_КШ."манчестер декодер ОС" ("Машина состояний КШ")) -> (s? t:f=w400:T2)
      }
      frame "чтение ОС" {
        # "Если флаг передачи - ложь,\nто ожидаем слова данных от ОУ."
        # "В этом ВП происходит\nчтение адреса ОУ, сравнивание\n с адресом этого ОУ. А так же\nрасчет и сравнение бита четности."
        # "17"
        n202 = local read "адрес ОУ (0-30)"() -> (w417:u8)
        n203 = call "Прием ОС (SubVI).vi"("Адрес ОУ"=w417, "RX Data"=w411) -> ("Ошибка ОС"=w407:bool)  [unwired: 8 in, 1 out]
        n204 = xnode ("Register Write")("Data"=w407) -> ()  [unwired: 1 in, 1 out]
        n205 = xnode ("Register Read")() -> ("Data"=w408:bool)  [unwired: 1 in, 1 out]
        n206 = Select(t=машина_состояний_КШ."ожидание команд" ("Машина состояний КШ"), s=w408, f=машина_состояний_КШ."ожидание rising СД" ("Машина состояний КШ")) -> (s? t:f=w416:T2)
      }
    }
    "Машина состояний КШ" <- w12
  }
  n207 = while {
    stop <- FALSE stop-if-true
    n208 = xnode "FPGA I/O Node"("ConnectorA/AO0"="Амплитуда (0-4096)") -> ()  [unwired: 1 in, 1 out]
  }
  n209 = node-c288(w1) -> ()
